vi "DriveMaxSpeed.vi"() -> (3 "Max Speed (ft/sec)":dbl)   [LabVIEW 2020]
doc: "Constant variable for max speed of robot to use in calculations"
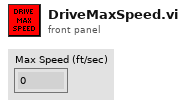
[diagram p1: front panel]
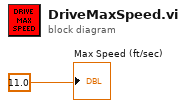
[diagram p0: block diagram]
diagram:
  "Max Speed (ft/sec)" <- 11.0
